vi "read all vision timestamps of files in a folder.vi"() -> ()   [LabVIEW 2020]
panel:
  out "XY Graph":cluster{i32[], dbl[]}(graph)
  out "Waveform Graph":dbl[](graph)
  in  "folder of camera device":path=path "\\\\192.168.13.6\\pdna2/data/Y2025/12-Dec/25_1208/scans/Scan028/CAM-HPD-CCD"
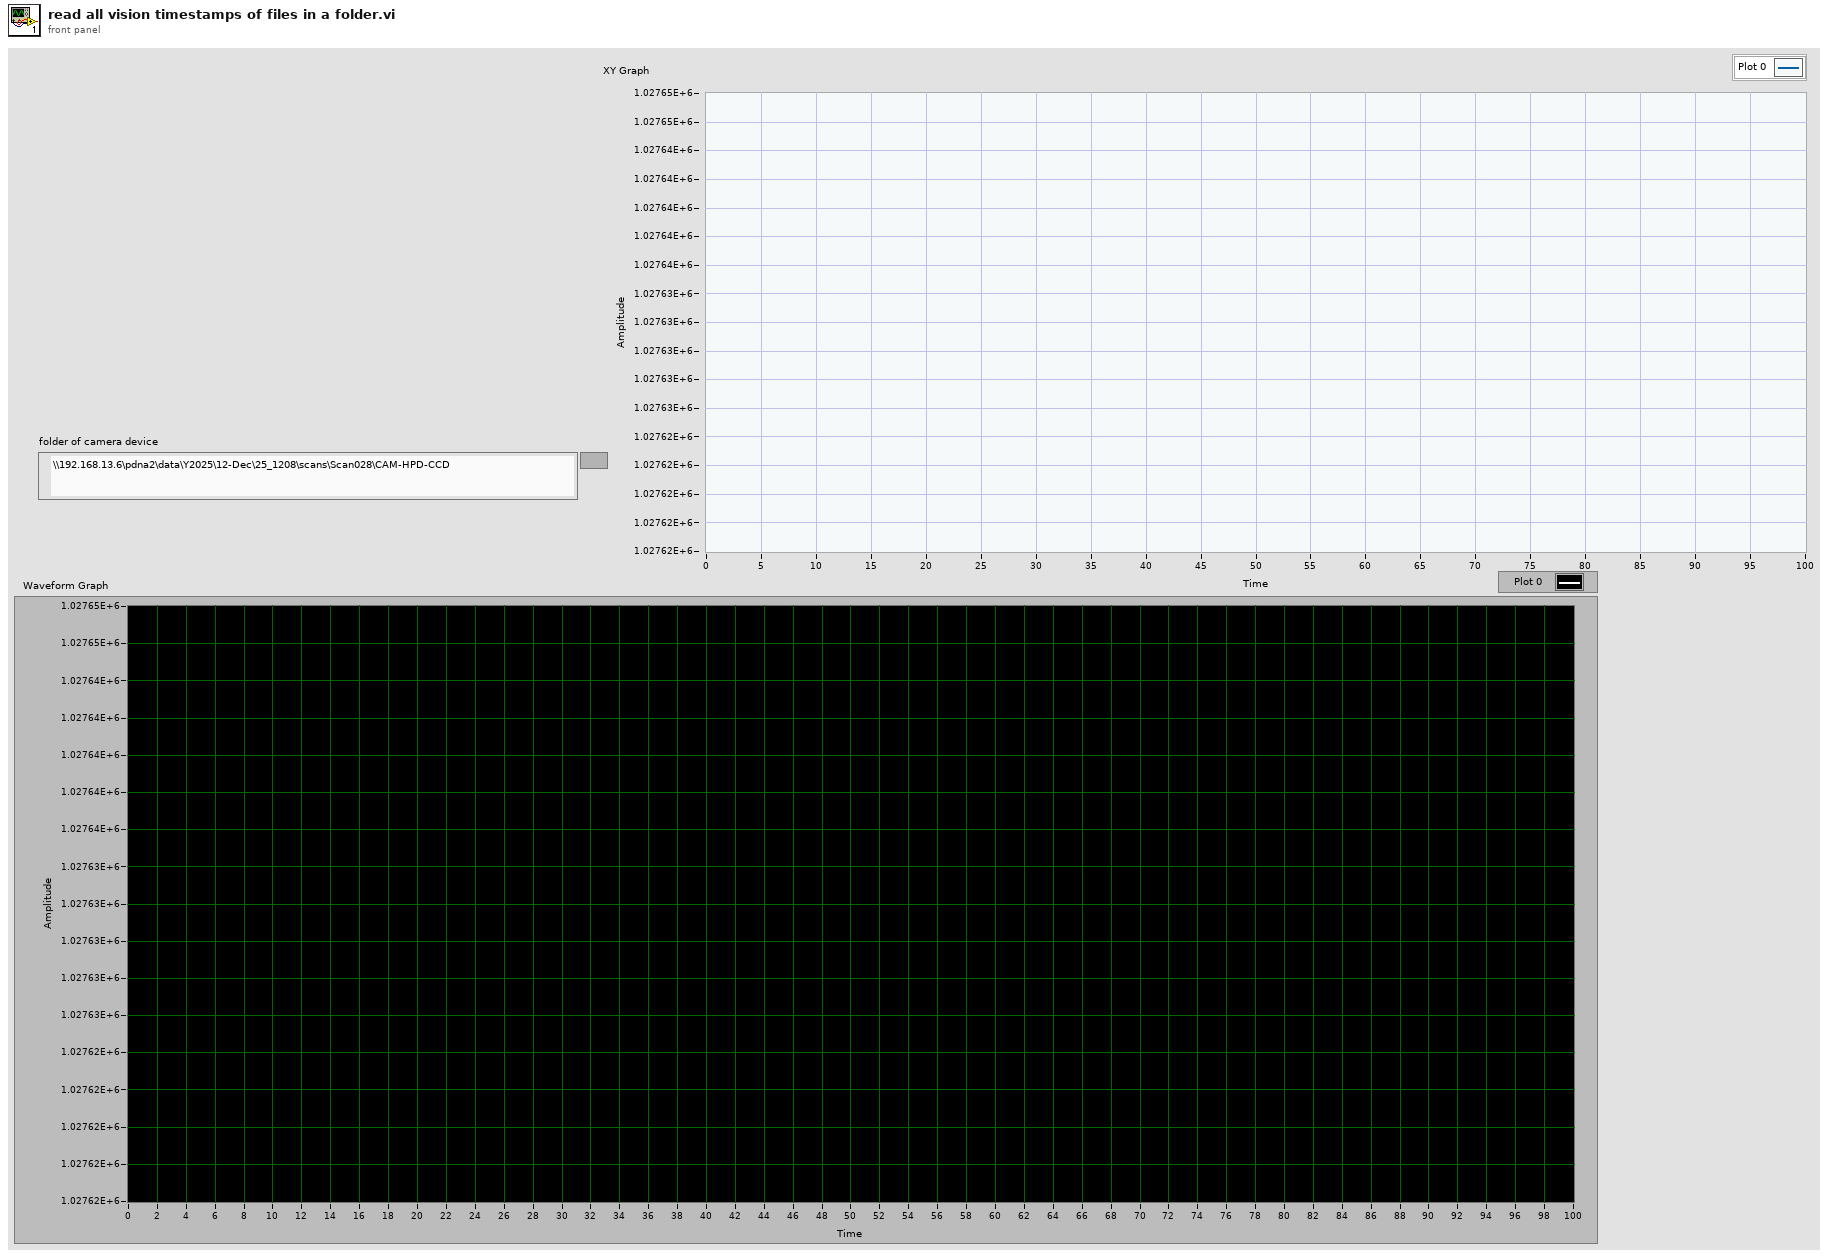
[diagram p1: front panel]
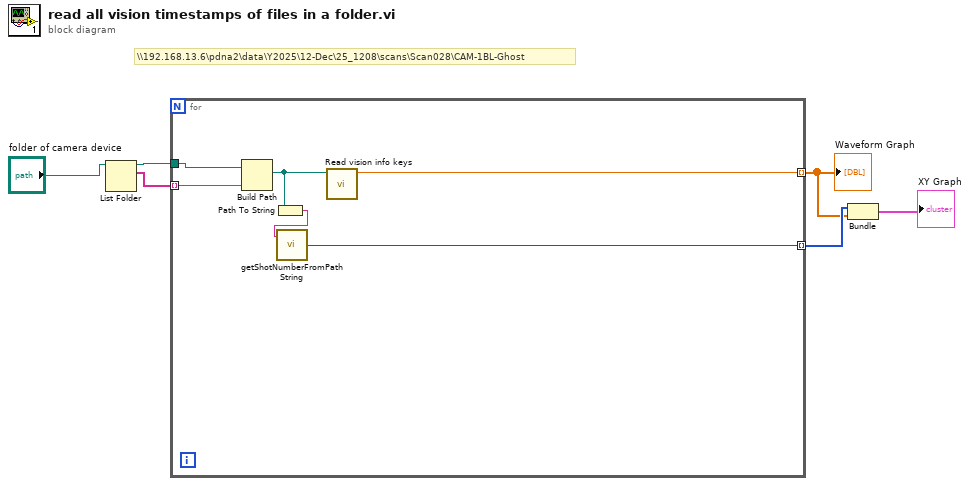
[diagram p0: block diagram]
diagram:
  # "\\\\192.168.13.6\\pdna2\\data\\Y2025\\12-Dec\\25_1208\\scans\\Scan028\\CAM-1BL-Ghost"
  n1 = List Folder(path="folder of camera device") -> (path out=w5:path, filenames=w4:string[])  [unwired: 3 in, 2 out]
  n2 = for {
    tunnel: w5 -> [w12]
    tunnel: w4 -> [w11] mode=indexing
    tunnel: [w10] -> w2 mode=indexing
    tunnel: [w7] -> w3 mode=indexing
    n3 = Build Path(base path=w12, name or relative path=w11) -> (appended path=w9:path)
    n4 = Path To String(path=w9) -> (string=w8:string)
    n5 = call "getShotNumberFromPathString.vi"("Path String"=w8) -> ("ShotNumber from path"=w7:i32)
    n6 = call "Read vision info keys.vi"("Image path"=w9) -> ("timestamp"=w10:dbl)  [unwired: 10 in]
  }
  "Waveform Graph" <- w2
  n7 = Bundle(w3, w2) -> (→"XY Graph":cluster{i32[], dbl[]})  [unwired: 1 in]
